vi "Read Output.vi"(8 "error in (no error)":errorcluster, 11 "Power Supply in":refnum<class "Power Supply.lvclass">) -> (0 "error out":errorcluster, 1 "persistent?":bool, 2 "Field":dbl[unit], 3 "Power Supply out":refnum<class "Power Supply.lvclass">, 4 "Power supply \"field\"":dbl[unit])   [LabVIEW 2012, in "Power Supply.lvclass"]
uses:
  Power Supply.lvclass
  Power Supply.lvclass/Power Supply.ctl
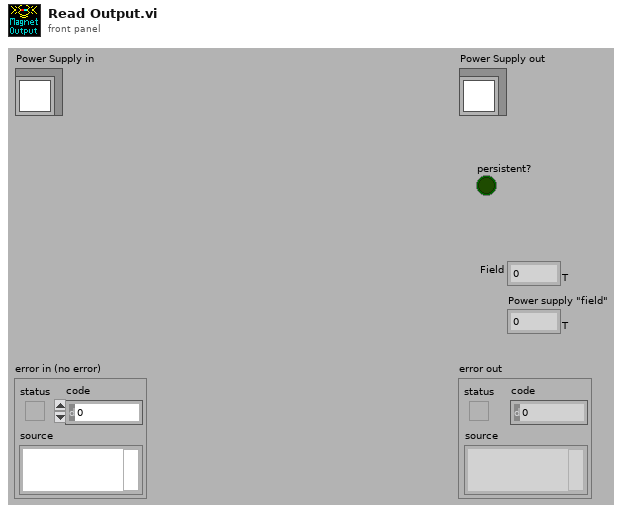
[diagram p1: front panel]
types:
  T1 = typedef "PSIO.ctl" = cluster{"Address":T2, "Version":enum16{"PS", "IPS"}}
  T2 = typedef "OxfordAddress.ctl" = cluster{"Com Port":i32, "ISOBUS Address":i32, "GPIB Address":i16, "Communication":enum16{"RS232", "ISOBUS", "GPIB", "Gateway"}}
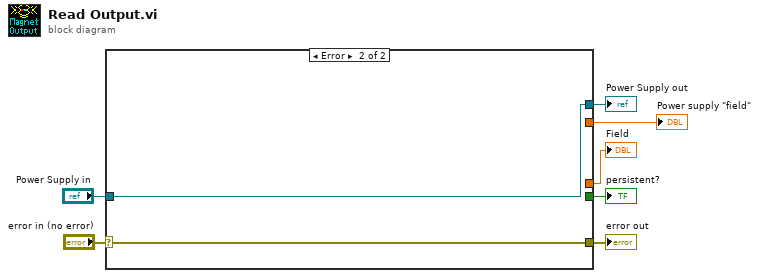
[diagram p0: block diagram]
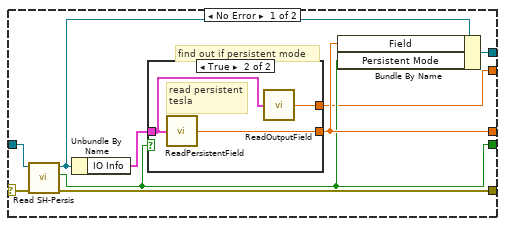
[diagram p2: hidden frame]
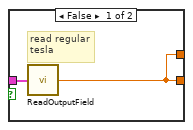
[diagram p3: hidden frame]
diagram:
  n1 = case shown="Error" "error in (no error)" {
    selector: "error in (no error)" -> [w12 w22]
    tunnel: [w9 _] -> w7
    tunnel: [w10 _] -> w6
    tunnel: "Power Supply in" -> [w16 w23]
    tunnel: [w15 w22] -> w4
    tunnel: [w11 w23] -> w3
    tunnel: [w8 _] -> w1
    frame No Error {
      # "find out if persistent mode"
      n2 = call-dynamic "Read SH-Persis.vi"("error in (no error)"=w12, "Power Supply in"=w16) -> ("error out"=w15:errorcluster, "pers?"=w9:bool, "Power Supply out"=w14:refnum<class "Power Supply.lvclass">)  [unwired: 4 in, 3 out]
      n3 = Unbundle By Name(w14) -> ("IO Info"=w13:T1)
      n4 = case shown="True" w9 {
        tunnel: w13 -> [w18 w20]
        tunnel: [w17 w21] -> w10
        tunnel: [w17 w19] -> w8
        frame False {
          # "read regular\ntesla"
          n5 = call "ReadOutputField.vi"("IO Info"=w18) -> ("Field"=w17:dbl[unit])  [unwired: 2 out]
        }
        frame True {
          # "read persistent\ntesla"
          n6 = call "ReadPersistentField.vi"("IO Info"=w20) -> ("Persistent Field"=w21:dbl[unit])  [unwired: 2 out]
          n7 = call "ReadOutputField.vi"("IO Info"=w20) -> ("Field"=w19:dbl[unit])  [unwired: 2 out]
        }
      }
      n8 = Bundle By Name(cluster=w14, "Field"=w10, "Persistent Mode"=w9) -> (w11:refnum<class "Power Supply.lvclass">)
    }
    frame Error {
    }
  }
  "persistent?" <- w7
  "Field" <- w6
  "Power Supply out" <- w3
  "error out" <- w4
  "Power supply \"field\"" <- w1
